vi "To More Specific Type (Boolean).vi"(8 "error in (no error)":errorcluster, 11 "JSON Datatype in":refnum<class "JSON Null.lvclass">) -> (0 "error out":errorcluster, 3 "JSON Datatype out":refnum<class "JSON Boolean.lvclass">)   [LabVIEW 2016, in "LVJSON.lvlib" / "JSON Helper.lvclass"]
doc: "Casts a JSON instance to the given JSON type"
uses:
  JSON Helper.lvclass
  JSON Datatype/JSON Null.lvclass
  JSON Boolean/JSON Boolean.lvclass
  Errors/Errors.ctl
  LVJSON.lvlib
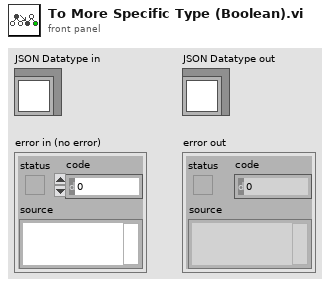
[diagram p1: front panel]
types:
  T1 = typedef "LVJSON.lvlib/Errors.ctl" = enum16{"No key", "Key path type", "Array OOB", "Type Mismatch", "Invalid Token"}
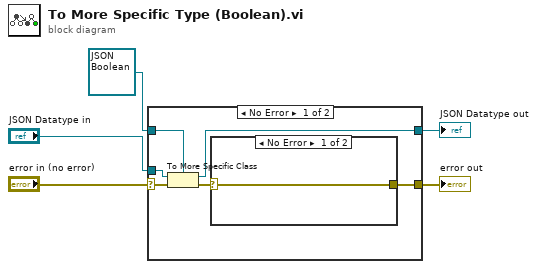
[diagram p0: block diagram]
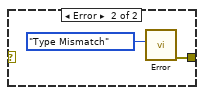
[diagram p2: hidden frame]
diagram:
  n1 = case shown="No Error" "error in (no error)" {
    selector: "error in (no error)" -> [w10 w16]
    tunnel: [w6 w16] -> w4
    tunnel: [w11 w15] -> w2
    tunnel: "JSON Datatype in" -> [w8 _]
    tunnel: refnum<class "JSON Boolean.lvclass"> refnum ("target class") -> [w9 w15]
    frame No Error {
      n2 = To More Specific Class(target class=w9, reference=w8, error in=w10) -> (specific class reference=w11:refnum<class "JSON Boolean.lvclass">, error out=w7:errorcluster)
      n3 = case shown="No Error" w7 {
        selector: w7 -> [w12 _]
        tunnel: [w12 w14] -> w6
        frame No Error {
        }
        frame Error {
          n4 = call "Error.vi"(9:Errors."Type Mismatch") -> ("error out"=w14:errorcluster)  [unwired: 9 in]
        }
      }
    }
    frame Error {
    }
  }
  "error out" <- w4
  "JSON Datatype out" <- w2
